vi "Write json to DOParam one.vi"(8 "error in (no error)":errorcluster, 10 "JSON Data In":string, 11 "DO in":T1) -> (0 "error out":errorcluster, 3 "DO out":T1)   [LabVIEW 2019, in "Inputs.lvlib"]
uses:
  Inputs.lvlib
  Ctl/DO.ctl
  Ctl/Parameter State.ctl
  Ctl/DOParamColumns.ctl
  <vilib>/JDP Science/JSONtext/Find Multiple Items.vi
  <vilib>/JDP Science/JSONtext/String Subset.vi
  <vilib>/JDP Science/JSONtext/support/Strip Quotes and Unescape.vi
  <vilib>/JDP Science/JSONtext/Parsing/Parse Full Path or Item Name.vi
  <vilib>/JDP Science/JSONtext/Offset/Find Item Locations by Path.vi
  <vilib>/JDP Science/JSONtext/support/Unescape JSON string.vi
  <vilib>/JDP Science/JSONtext/Get Array Elements.vi
  Userlib.lvlib
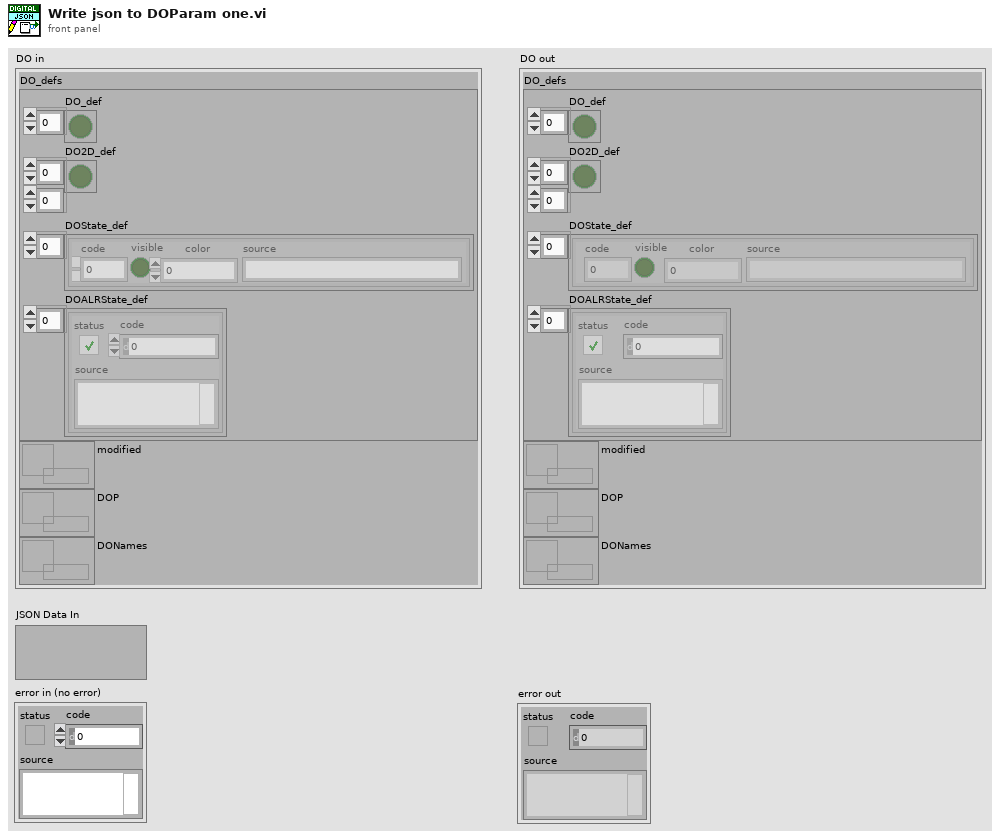
[diagram p1: front panel]
types:
  T1 = typedef "Inputs.lvlib/DO.ctl" = cluster{"DO_defs":cluster{"DO_def":bool[], "DO2D_def":bool[][], "DOState_def":T2[], "DOALRState_def":errorcluster[]}, "modified":refnum<data-value>, "DOP":refnum<data-value>, "DONames":refnum<data-value>}
  T2 = typedef "Inputs.lvlib/Parameter State.ctl" = cluster{"code":i32, "visible":bool, "color":u32, "source":string}
  T3 = typedef "Inputs.lvlib/DOParamColumns.ctl" = enum16{"module_fcode_full", "control_channel_num", "fcode", "fcodef", "fcode_full", "fname"}
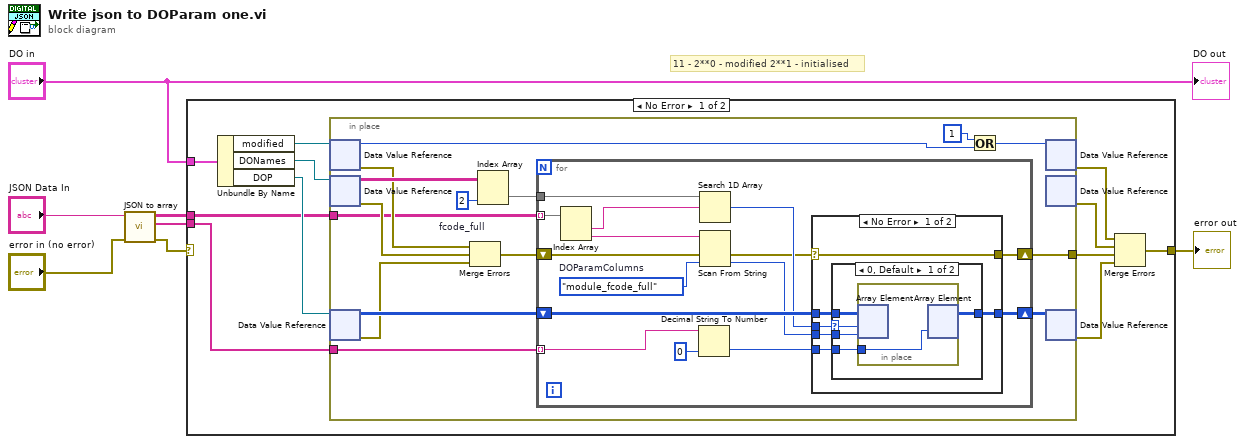
[diagram p0: block diagram]
diagram:
  # "11 - 2**0 - modified 2**1 - initialised"
  n1 = call "JSON to array.vi"("error in (no error)"="error in (no error)", "JSON Data In"="JSON Data In") -> ("error out"=w4:errorcluster, "values"=w1:string[], "names"=w2:string[][])  [unwired: 7 in]
  n2 = case shown="No Error" w4 {
    selector: w4 -> [_ w64]
    tunnel: [w17 w64] -> w7
    tunnel: "DO in" -> [w18 _]
    tunnel: w1 -> [w15 _]
    tunnel: w2 -> [w10 _]
    frame No Error {
      n3 = Unbundle By Name(w18) -> ("modified"=w12:refnum<data-value>, "DONames"=w14:refnum<data-value>, "DOP"=w16:refnum<data-value>)
      n4 = in-place {
        in-place-border: w15 -> [w25]
        in-place-border: [w26] -> w8
        in-place-border: w10 -> [w19]
        w30 = 2  # fcode_full
        n5 = in-place-dvr #1(w12) -> (w23:u8, w21:errorcluster)
        n6 = in-place-dvr #2(w14) -> (w31:string[][], w28:errorcluster)
        n7 = in-place-dvr #3(w16) -> (w33:i32[][], w27:errorcluster)
        n8 = Merge Errors(w21, w28, w27) -> (w20:errorcluster)
        n9 = Index Array(array=w31, index (col)=w30) -> (element=w29:string[])  [unwired: 1 in]
        n10 = for {
          tunnel: w29 -> [w46]
          tunnel: w25 -> [w41] mode=indexing
          shift-right: [w42] -> w26
          shift-left: w20 -> [w38]
          shift-right: [w47] -> w32
          shift-left: w33 -> [w48]
          tunnel: w19 -> [w36] mode=indexing
          w45 = DOParamColumns."module_fcode_full"  # DOParamColumns
          n11 = Index Array(array=w36) -> (element #1=w35:string, element #2=w34:string)  [unwired: 2 in]
          n12 = Decimal String To Number(string=w41, default (0L)=0 ("default (0 DBL)")) -> (number=w40:i32)  [unwired: 1 in, 1 out]
          n13 = Search 1D Array(1D array=w46, element=w35) -> (index of element=w44:i32)  [unwired: 1 in]
          n14 = Scan From String(input string=w34, error in=w38, default 1=w45) -> (error out=w37:errorcluster, output 1=w43:T3)  [unwired: 2 in, 2 out]
          n15 = case shown="No Error" w37 {
            selector: w37 -> [w49 w62]
            tunnel: w48 -> [w54 w63]
            tunnel: [w53 w63] -> w47
            tunnel: w43 -> [w52 _]
            tunnel: w40 -> [w51 _]
            tunnel: w44 -> [w50 _]
            tunnel: [w49 w62] -> w42
            frame No Error {
              n16 = case shown="0, Default" w50 {
                selector: w50 -> [w55 _]
                tunnel: w54 -> [w59 w61]
                tunnel: [w58 w61] -> w53
                tunnel: w52 -> [w57 _]
                tunnel: w51 -> [w56 _]
                frame 0, Default {
                  n17 = in-place {
                    in-place-border: w56 -> [w60]
                    n18 = in-place-array #4(w59, w55, w57) -> ()  [unwired: 1 out]
                    n19 = in-place-array #4(w60) -> (w58:i32[][])  [unwired: 2 out]
                  }
                }
                frame -1 {
                }
              }
            }
            frame Error {
            }
          }
        }
        n20 = Or(x=u8 1 ("data value"), y=w23) -> (x .or. y?=w22:u8)
        n21 = in-place-dvr #1(w22) -> (w11:errorcluster)  [unwired: 1 out]
        n22 = in-place-dvr #2() -> (w13:errorcluster)  [unwired: 1 in, 1 out]
        n23 = in-place-dvr #3(w32) -> (w9:errorcluster)  [unwired: 1 out]
      }
      n24 = Merge Errors(w11, w13, w8, w9) -> (w17:errorcluster)
    }
    frame Error {
    }
  }
  "error out" <- w7
  "DO out" <- "DO in"
